vi "LEBITVacuum.TrendMessage.vi"(0 "i ref in":refnum<vi>, 1 "data":i16, 2 "i attribute":T1={"setValuePLC"=[], "nickNames"=[], "setValuePLCServiceID"=[], "monValuePLC"=[], "SetValueServiceID"=[], "MonValueServiceID"=[], "SetValue"=[], "AllPLCValues"=[], "CondSpecial2DArray"=[], "CondSpecialIndex"=[], "ReasonForLocking"="", "ReasonForLockingID"=0, "enableValuePLC"=[], "OverwriteCloseSafetyPLC"=[], "OverwriteOpenSafetyPLC"=[], "OverwriteCloseSafetyPLCServiceID"=[], "OverwriteOpenSafetyPLCServiceID"=[], "MKS Address Array"=[], "MKS MeasurementServiceID"=[], "MKS Measurement"=[], "CRYO Measurement"=[], "CRYO MeasurementServiceID"=[], "Special"=[], "Start Date"="", "MKS VISA resource"="COM13", "CRYO VISA resource"="COM13"}, 3 "index":i32, 5 "error in":errorcluster, 6 "quality":i32, 9 "no link":bool) -> (14 "i ref out":refnum<vi>, 16 "i attribute out":T1={"setValuePLC"=[], "nickNames"=[], "setValuePLCServiceID"=[], "monValuePLC"=[], "SetValueServiceID"=[], "MonValueServiceID"=[], "SetValue"=[], "AllPLCValues"=[], "CondSpecial2DArray"=[], "CondSpecialIndex"=[], "ReasonForLocking"="", "ReasonForLockingID"=0, "enableValuePLC"=[], "OverwriteCloseSafetyPLC"=[], "OverwriteOpenSafetyPLC"=[], "OverwriteCloseSafetyPLCServiceID"=[], "OverwriteOpenSafetyPLCServiceID"=[], "MKS Address Array"=[], "MKS MeasurementServiceID"=[], "MKS Measurement"=[], "CRYO Measurement"=[], "CRYO MeasurementServiceID"=[], "Special"=[], "Start Date"="", "MKS VISA resource"="COM13", "CRYO VISA resource"="COM13"}, 17 "Is Off?":bool, 19 "error out":errorcluster)   [LabVIEW 2014, in "LEBITVacuum.lvlib"]
uses:
  LEBITVacuum.lvlib
  LEBITVacuum.i attribute.ctl
  CSlibraries/UtilityLib/UtilityLib.valueStatus.ctl
  CSlibraries-extern/DimLVEvent/LVDimInterface/LVDimInterface.lvlib
  CSlibraries/UtilityLib/UtilityLib.lvlib
  CSCore/CSSystem/CoreLib/CoreLib.lvlib
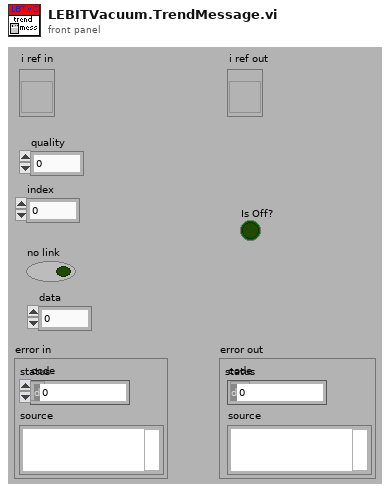
[diagram p1: front panel]
types:
  T1 = typedef "LEBITVacuum.lvlib/LEBITVacuum.i attribute.ctl" = cluster{"setValuePLC":string[], "nickNames":string[], "setValuePLCServiceID":i32[], "monValuePLC":string[], "SetValueServiceID":i32[], "MonValueServiceID":i32[], "SetValue":i16[], "AllPLCValues":string[], "CondSpecial2DArray":string[][], "CondSpecialIndex":i32[], "ReasonForLocking":string, "ReasonForLockingID":i32, "enableValuePLC":string[], "OverwriteCloseSafetyPLC":string[], "OverwriteOpenSafetyPLC":string[], "OverwriteCloseSafetyPLCServiceID":i32[], "OverwriteOpenSafetyPLCServiceID":i32[], "MKS Address Array":i32[][], "MKS MeasurementServiceID":i32[], "MKS Measurement":string[], "CRYO Measurement":string[][], "CRYO MeasurementServiceID":i32[], "Special":string[], "Start Date":string, "MKS VISA resource":refnum<visa-resource-name>, "CRYO VISA resource":refnum<visa-resource-name>}
  T2 = typedef "UtilityLib.lvlib/UtilityLib.valueStatus.ctl" = enum16{"no info available", "stand by/off", "on", "warning", "alarm/malfunction", "not implemented", "user action required", "important information", "system default", "control default", "indicator default", "button default"}
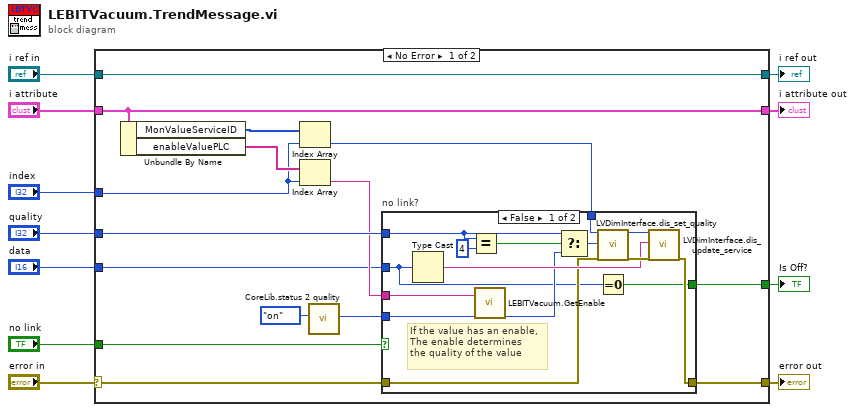
[diagram p0: block diagram]
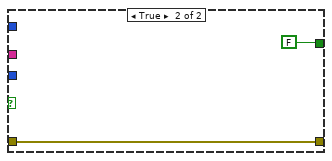
[diagram p2: hidden frame]
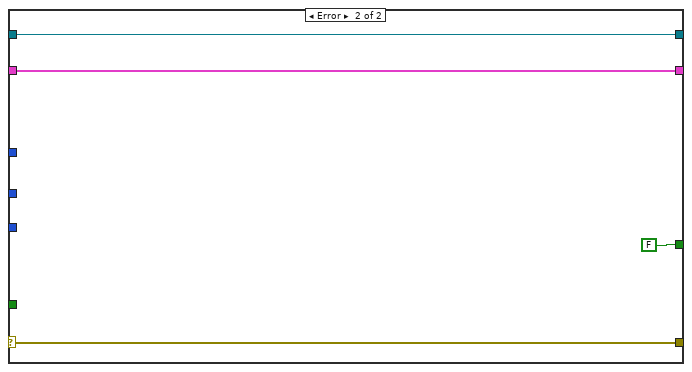
[diagram p3: hidden frame]
diagram:
  n1 = case shown="No Error" "error in" {
    selector: "error in" -> [w13 w47]
    tunnel: "quality" -> [w26 _]
    tunnel: "no link" -> [w25 _]
    tunnel: [w22 w47] -> w9
    tunnel: "data" -> [w14 _]
    tunnel: "i attribute" -> [w21 w45]
    tunnel: "i ref in" -> [w20 w46]
    tunnel: [w20 w46] -> w5
    tunnel: "index" -> [w15 _]
    tunnel: [w21 w45] -> w3
    tunnel: [w12 FALSE] -> w1
    frame No Error {
      n2 = Unbundle By Name(w21) -> ("MonValueServiceID"=w16:i32[], "enableValuePLC"=w18:string[])
      n3 = Index Array(array=w16, index=w15) -> (element=w23:i32)
      n4 = Index Array(array=w18, index=w15) -> (element=w17:string)
      n5 = call "CoreLib.status 2 quality.vi"("valueStatus"=UtilityLib.valueStatus."on") -> ("quality"=w24:i32)  [unwired: 18 in]
      n6 = case "no link?" shown="False" w25 {
        tunnel: w14 -> [w27 _]
        tunnel: w26 -> [w33 _]
        tunnel: w24 -> [w31 _]
        tunnel: w23 -> [w39 _]
        tunnel: [w36 w43] -> w22
        tunnel: w17 -> [w30 _]
        tunnel: w13 -> [w29 w43]
        tunnel: [w28 FALSE] -> w12
        frame False {
          # "If the value has an enable,\nThe enable determines\nthe quality of the value"
          n7 = Type Cast(x=w27) -> (*(type *) &x=w37:string)  [unwired: 1 in]
          n8 = Equal?(x=w33, y=4) -> (x = y?=w34:bool)
          n9 = call "LEBITVacuum.GetEnable.vi"("EnableValuePLC"=w30, "quality in"=w31) -> ("quality out"=w32:i32)  [unwired: 17 in]
          n10 = Select(t=w33, s=w34, f=w32) -> (s? t:f=w40:i32)
          n11 = call "LVDimInterface.dis_set_quality.vi"("my_serviceID"=w39, "quality"=w40, "error in (no error)"=w29) -> ("my_serviceID (out)"=w38:i32, "error out"=w41:errorcluster)  [unwired: 15 in]
          n12 = Equal To 0?(x=w27) -> (x = 0?=w28:bool)
          n13 = call "LVDimInterface.dis_update_service.vi"("my_serviceID"=w38, "data"=w37, "error in (no error)"=w41) -> ("error out"=w36:errorcluster)  [unwired: 14 in, 2 out]
        }
        frame True {
        }
      }
    }
    frame Error {
    }
  }
  "error out" <- w9
  "i ref out" <- w5
  "i attribute out" <- w3
  "Is Off?" <- w1
